vi "Get Section Scalars.vi"(8 "error in":errorcluster, 11 "section ref in":T1 format="%.0x") -> (0 "error out":errorcluster, 2 "section scalars out":T2[](array[typedef]), 3 "section ref in":T1 format="%.0x")   [LabVIEW 2019, in "Scripting API.lvlib"]
uses:
  Scripting API.lvlib
  <vilib>/NI VeriStand/Custom Device API/Custom Device Item Ref.ctl
  TypeDefs/Output Scalar Data.ctl
  Addon/Addon Shared/Types/FPGA Addon Data Type.ctl
  Addon/Addon Shared/Types/FG Action.ctl
  Addon/Addon Shared/Types/Register Information.ctl
  Addon/Addon Shared/SubVIs/Constants.vi
  <vilib>/NI/NI VeriStand Advanced SysDef API/SysDef API/SysDef.Property.Get.vi
  <vilib>/NI/NI VeriStand Advanced SysDef API/_SubVIs/SysDef.Property.Get.Variant.vi
  <vilib>/NI/NI VeriStand Advanced SysDef API/SysDef API/SysDef.Property.Set.vi
  <vilib>/NI/NI VeriStand Advanced SysDef API/_SubVIs/SysDef.Property.Set.Variant.vi
  Addon/Addon Shared/FPGA Addon Shared.lvlib
  <vilib>/NI VeriStand/Custom Device API/Custom Device API.lvlib
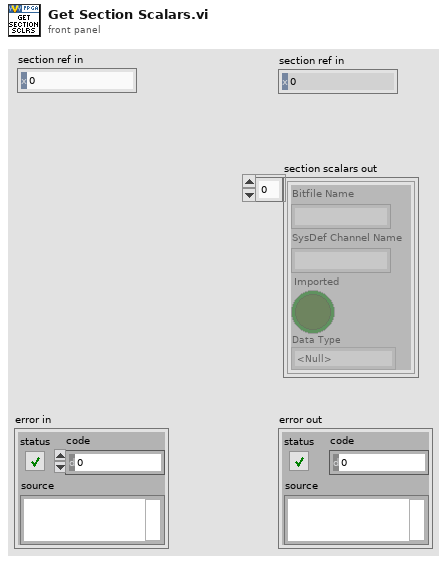
[diagram p1: front panel]
types:
  T1 = typedef "Custom Device API.lvlib/Custom Device Item Ref.ctl" = u64
  T2 = typedef "Scripting API.lvlib/Output Scalar Data.ctl" = cluster{"Bitfile Name":string, "SysDef Channel Name":string, "Imported":bool, "Data Type":T3}
  T3 = typedef "FPGA Addon Shared.lvlib/FPGA Addon Data Type.ctl" = enum8{"<Null>", "I8", "I16", "I32", "I64", "U8", "U16", "U32", "U64", "SGL", "Boolean", "Analog PWM In Settings", "Analog PWM In", "Digital PWM In Settings", "Digital PWM In", "Digital PWM Out", "Sine Out", "FXP", "FXP+/-24.5", "FXP+/-16.5", "FXP+/-32.8", "FXP+/-64.32", "FXP+/-16.7", "FXP+/-20.5", "FXP+/-27.5", "FXP+/-32.16", "FXP+16.3", "FXP+18.3", "Digital Static In", "Digital Static Out", "Digital Static In Settings", "Digital WSS Out", "Quad Encoder Settings", "Quad Encoder In", "Group"}
  T4 = typedef "FPGA Addon Shared.lvlib/FG Action.ctl" = enum8{"GET", "SET"}
  T5 = typedef "FPGA Addon Shared.lvlib/Register Information.ctl" = cluster{"Name":string, "Data Type":T3, "Default Value":variant, "Attributes":variant}
  T6 = typedef "Custom Device API.lvlib/Custom Device Item Info.ctl" = cluster{"Name":string, "Is Channel":bool, "GUID":string, "Is Waveform":bool}
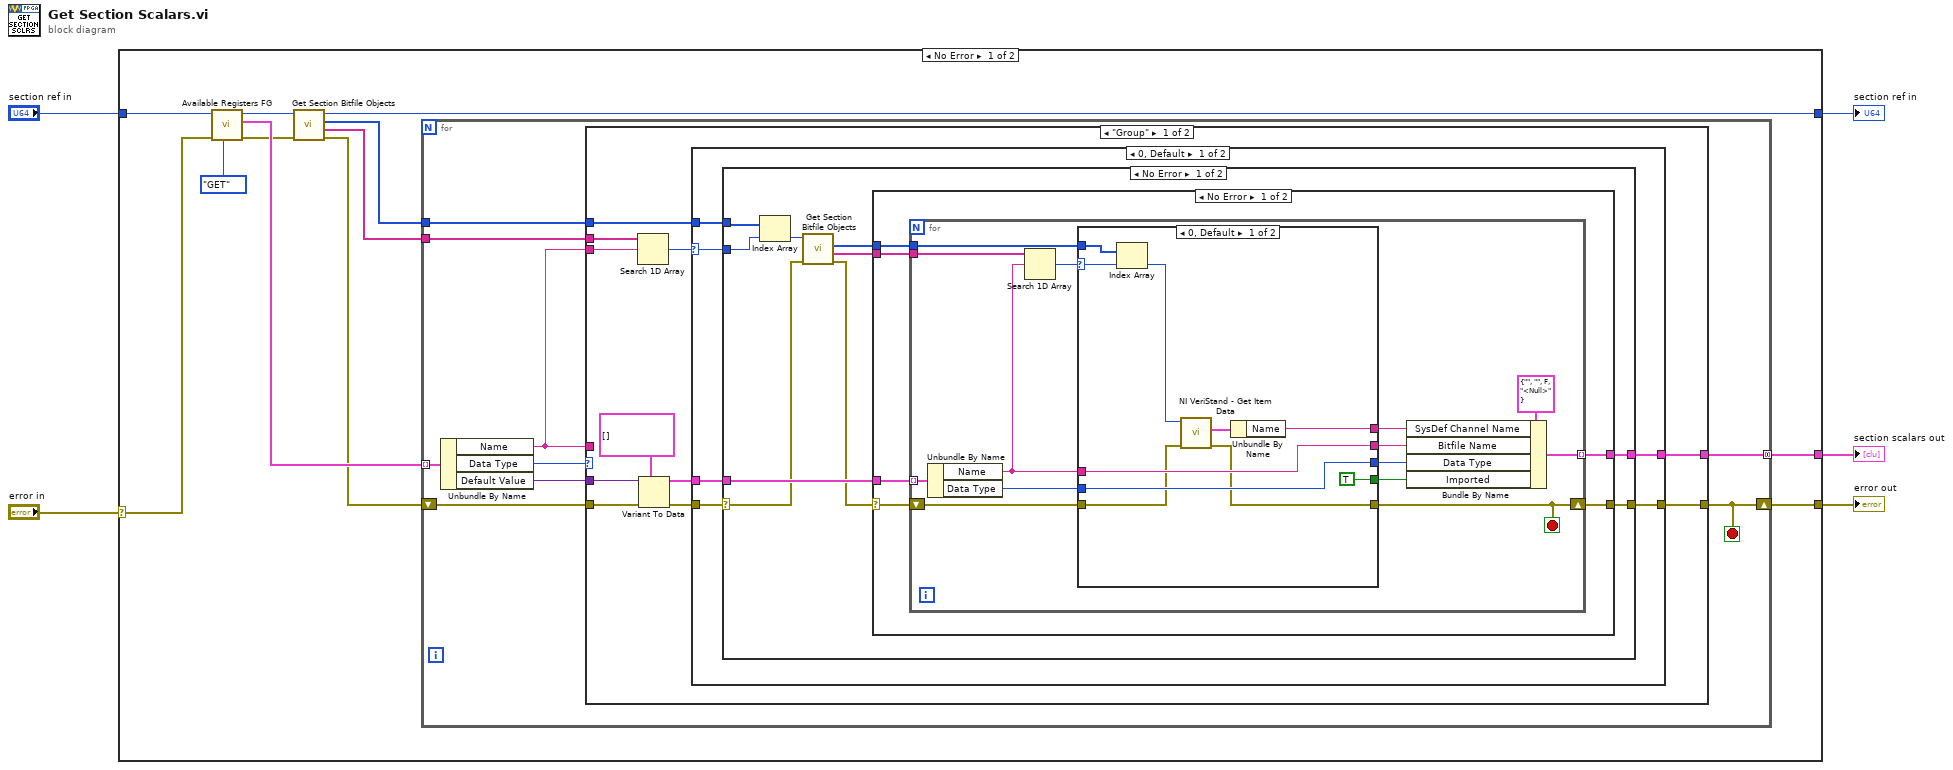
[diagram p0: block diagram]
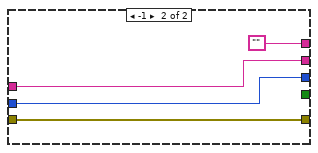
[diagram p2: hidden frame]
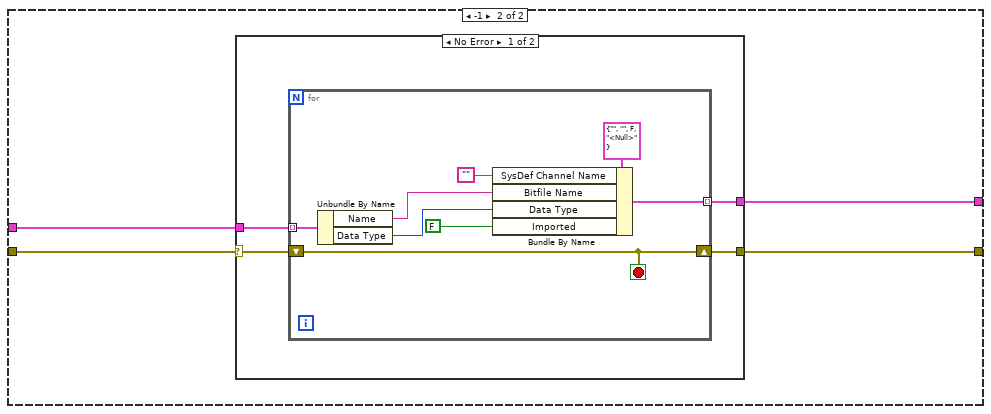
[diagram p5: hidden frame]
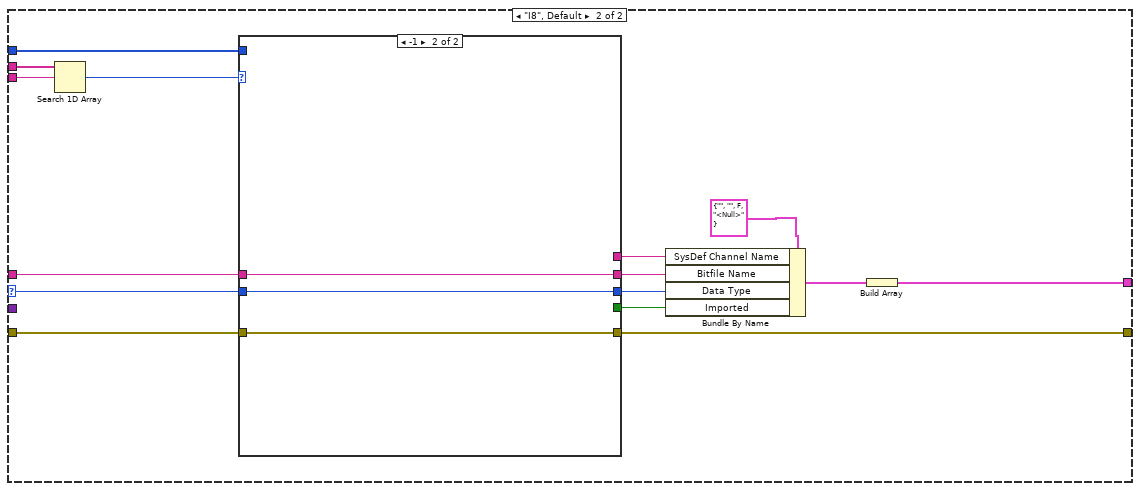
[diagram p7: hidden frame]
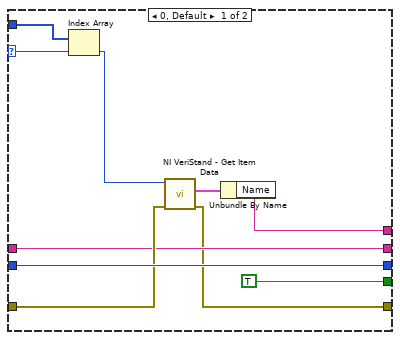
[diagram p8: hidden frame]
diagram:
  n1 = case shown="No Error" "error in" {
    selector: "error in" -> [w8 w136]
    tunnel: "section ref in" -> [w15 w135]
    tunnel: [w7 w135] -> w4
    tunnel: [w10 w136] -> w2
    tunnel: [w9 _] -> w1
    frame No Error {
      n2 = call "Available Registers FG.vi"("Action"=FG_Action."GET", "error in (no error)"=w8, "Item Ref"=w15) -> ("error out"=w12:errorcluster, "Available Registers"=w17:T5[], "Item Ref out"=w16:T1)  [unwired: 6 in]
      n3 = call "Get Section Bitfile Objects.vi"("error in"=w12, "item ref in"=w16) -> ("error out"=w11:errorcluster, "bitfile object names"=w13:string[], "section children refs"=w6:T1[], "item ref out"=w7:T1)  [unwired: 6 in]
      n4 = for {
        tunnel: w13 -> [w23]
        tunnel: w17 -> [w26] mode=indexing
        shift-right: [w18] -> w10
        shift-left: w11 -> [w21]
        tunnel: w6 -> [w24]
        tunnel: [w19] -> w9 mode=concatenating
        stop <- w18 stop-if-true
        n5 = Unbundle By Name(w26) -> ("Name"=w22:string, "Data Type"=w25:T3, "Default Value"=w20:variant)
        n6 = case shown="\"Group\"" w25 {
          selector: w25 -> [_ w113]
          tunnel: w24 -> [w30 w118]
          tunnel: w22 -> [w31 w121]
          tunnel: w23 -> [w32 w120]
          tunnel: w22 -> [_ w117]
          tunnel: w21 -> [w37 w112]
          tunnel: [w29 w109] -> w18
          tunnel: w20 -> [w36 _]
          tunnel: [w28 w107] -> w19
          frame "Group" {
            n7 = Search 1D Array(1D array=w32, element=w31) -> (index of element=w27:i32)  [unwired: 1 in]
            n8 = Variant To Data(error in=w37, type=T5[] [], Variant=w36) -> (data=w34:T5[], error out=w33:errorcluster)
            n9 = case shown="0, Default" w27 {
              selector: w27 -> [w38 _]
              tunnel: w34 -> [w43 w93]
              tunnel: w33 -> [w42 w90]
              tunnel: w30 -> [w41 _]
              tunnel: [w40 w91] -> w29
              tunnel: [w39 w92] -> w28
              frame 0, Default {
                n10 = case shown="No Error" w42 {
                  selector: w42 -> [w45 w89]
                  tunnel: w43 -> [w53 _]
                  tunnel: w41 -> [w52 _]
                  tunnel: w38 -> [w51 _]
                  tunnel: [w47 w89] -> w40
                  tunnel: [w46 _] -> w39
                  frame No Error {
                    n11 = Index Array(array=w52, index=w51) -> (element=w50:T1)
                    n12 = call "Get Section Bitfile Objects.vi"("error in"=w45, "item ref in"=w50) -> ("error out"=w44:errorcluster, "bitfile object names"=w49:string[], "section children refs"=w48:T1[])  [unwired: 6 in, 1 out]
                    n13 = case shown="No Error" w44 {
                      selector: w44 -> [w54 w88]
                      tunnel: w53 -> [w59 _]
                      tunnel: w49 -> [w58 _]
                      tunnel: w48 -> [w57 _]
                      tunnel: [w56 w88] -> w47
                      tunnel: [w55 _] -> w46
                      frame No Error {
                        n14 = for {
                          tunnel: w59 -> [w73] mode=indexing
                          tunnel: w58 -> [w72]
                          tunnel: w57 -> [w61]
                          shift-right: [w62] -> w56
                          shift-left: w54 -> [w65]
                          tunnel: [w63] -> w55 mode=indexing
                          stop <- w62 stop-if-true
                          n15 = Unbundle By Name(w73) -> ("Name"=w69:string, "Data Type"=w71:T3)
                          n16 = Search 1D Array(1D array=w72, element=w69) -> (index of element=w60:i32)  [unwired: 1 in]
                          n17 = case shown="0, Default" w60 {
                            selector: w60 -> [w74 _]
                            tunnel: w71 -> [w81 w86]
                            tunnel: w69 -> [w82 w87]
                            tunnel: [w82 w87] -> w68
                            tunnel: [w81 w86] -> w67
                            tunnel: [TRUE ("Imported?") _] -> w66
                            tunnel: w65 -> [w79 w85]
                            tunnel: [w78 ""] -> w64
                            tunnel: [w77 w85] -> w62
                            tunnel: w61 -> [w76 _]
                            frame 0, Default {
                              n18 = Index Array(array=w76, index=w74) -> (element=w75:T1)
                              n19 = call <vilib>:"NI VeriStand - Get Item Data.vi"("error in (no error)"=w79, "Item Ref in"=w75) -> ("error out"=w77:errorcluster, "Item Info"=w83:T6)  [unwired: 6 in, 2 out]
                              n20 = Unbundle By Name(w83) -> ("Name"=w78:string)
                            }
                            frame -1 {
                            }
                          }
                          n21 = Bundle By Name(cluster=T2 {"Bitfile Name"="", "SysDef Channel Name"="", "Imported"=FALSE, "Data Type"=enum."<Null>"} ("Scalar data"), "SysDef Channel Name"=w64, "Bitfile Name"=w68, "Data Type"=w67, "Imported"=w66) -> (w63:T2)
                        }
                      }
                      frame Error {
                      }
                    }
                  }
                  frame Error {
                  }
                }
              }
              frame -1 {
                n22 = case shown="No Error" w90 {
                  selector: w90 -> [w94 w106]
                  tunnel: w93 -> [w97 _]
                  tunnel: [w96 _] -> w92
                  tunnel: [w95 w106] -> w91
                  frame No Error {
                    n23 = for {
                      tunnel: w97 -> [w105] mode=indexing
                      shift-right: [w99] -> w95
                      shift-left: w94 -> [w99]
                      tunnel: [w100] -> w96 mode=indexing
                      stop <- w99 stop-if-true
                      n24 = Unbundle By Name(w105) -> ("Name"=w103:string, "Data Type"=w102:T3)
                      n25 = Bundle By Name(cluster=T2 {"Bitfile Name"="", "SysDef Channel Name"="", "Imported"=FALSE, "Data Type"=enum."<Null>"} ("Scalar data"), "SysDef Channel Name"="", "Bitfile Name"=w103, "Data Type"=w102, "Imported"=FALSE ("Imported?")) -> (w100:T2)
                    }
                  }
                  frame Error {
                  }
                }
              }
            }
          }
          frame "I8", Default {
            n26 = Search 1D Array(1D array=w120, element=w121) -> (index of element=w119:i32)  [unwired: 1 in]
            n27 = case shown="-1" w119 {
              selector: w119 -> [w130 _]
              tunnel: w118 -> [w131 _]
              tunnel: w117 -> [w123 w134]
              tunnel: [w127 _] -> w115
              tunnel: [w126 w133] -> w114
              tunnel: w113 -> [w126 w133]
              tunnel: w112 -> [w125 w132]
              tunnel: [TRUE _] -> w111
              tunnel: [w123 w134] -> w110
              tunnel: [w122 w132] -> w109
              frame 0, Default {
                n28 = Index Array(array=w131, index=w130) -> (element=w129:T1)
                n29 = call <vilib>:"NI VeriStand - Get Item Data.vi"("error in (no error)"=w125, "Item Ref in"=w129) -> ("error out"=w122:errorcluster, "Item Info"=w128:T6)  [unwired: 6 in, 2 out]
                n30 = Unbundle By Name(w128) -> ("Name"=w127:string)
              }
              frame -1 {
              }
            }
            n31 = Bundle By Name(cluster=T2 {"Bitfile Name"="", "SysDef Channel Name"="", "Imported"=FALSE, "Data Type"=enum."<Null>"} ("Scalar data"), "SysDef Channel Name"=w115, "Bitfile Name"=w110, "Data Type"=w114, "Imported"=w111) -> (w108:T2)
            n32 = Build Array(w108) -> (w107:T2[])
          }
        }
      }
    }
    frame Error {
    }
  }
  "section scalars out" <- w1
  "section ref in" <- w4
  "error out" <- w2
